vi "Search#OfTest.vi"(8 "TestStatusPath":path, 11 "MatchedSerialNumber":string) -> (3 "#OfTest":i32)   [LabVIEW 2011]
panel:
  out "#OfTest":string
  out "Status":string
  out "DateTime":string
  out "SerialNumber":string
  out "text":string
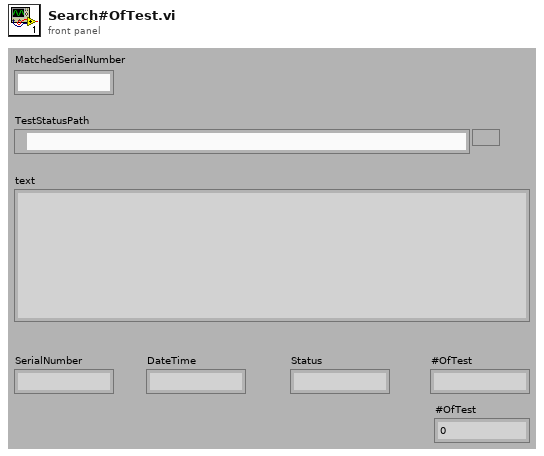
[diagram p1: front panel]
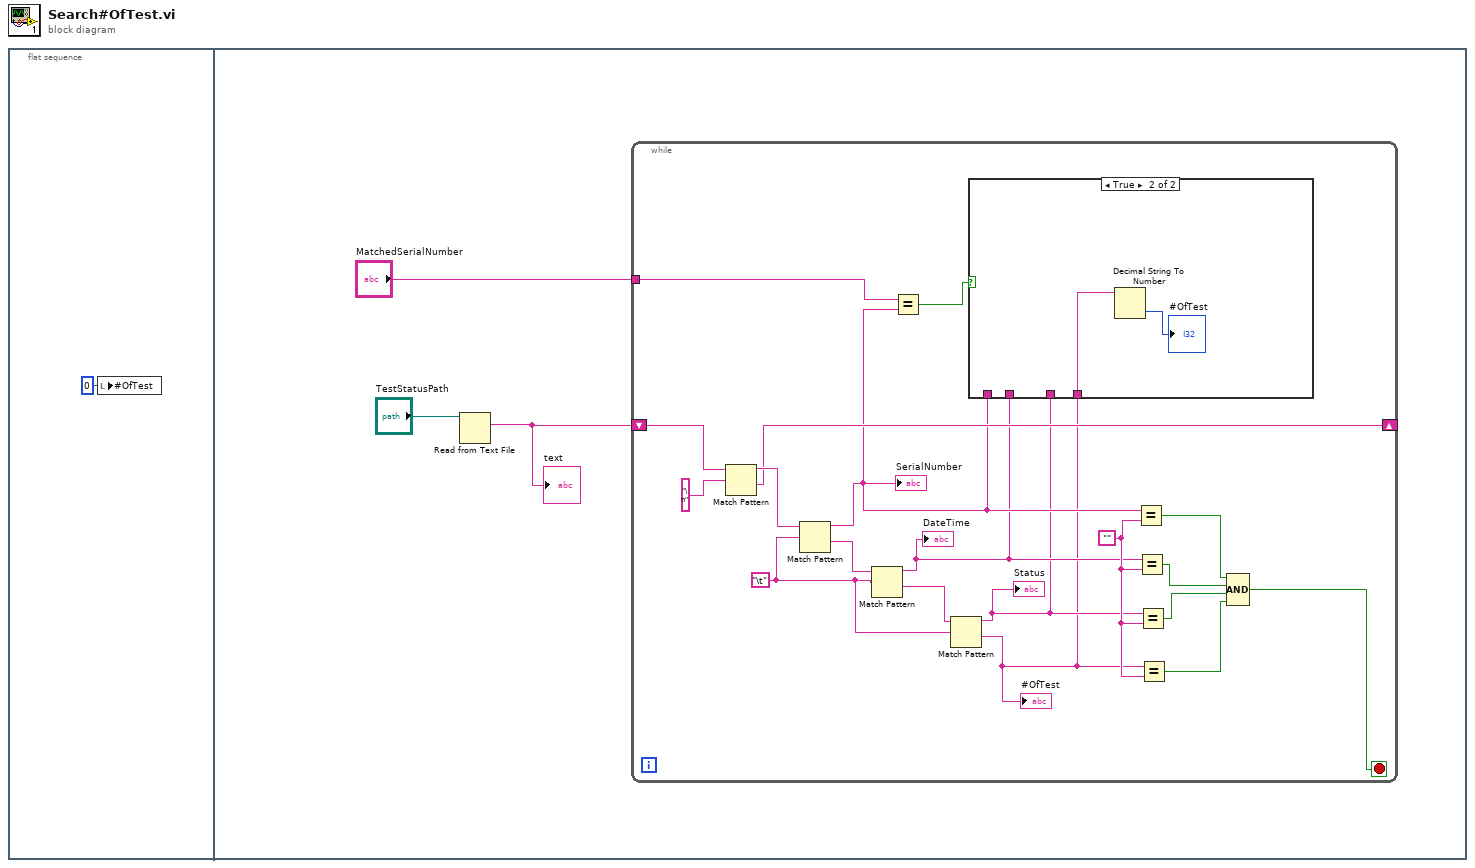
[diagram p0: block diagram]
diagram:
  n1 = flat-sequence {
    frame #0 {
      n2 = local write "#OfTest"(0 ("#OfTest")) -> ()
    }
    frame #1 {
      n3 = Read from Text File(file (use dialog)="TestStatusPath") -> (text=w4:string)  [unwired: 1 in, 5 out]
      "text" <- w4
      n4 = while {
        shift-right: [w11] -> _
        shift-left: w4 -> [w23]
        tunnel: "MatchedSerialNumber" -> [w10]
        stop <- w13 stop-if-true
        w18 = ""
        w19 = "\t"
        n5 = Match Pattern(string=w23, regular expression="\n") -> (before substring=w12:string, after substring=w11:string)  [unwired: 3 out]
        n6 = Match Pattern(string=w12, regular expression=w19) -> (before substring=w8:string, after substring=w21:string)  [unwired: 3 out]
        "SerialNumber" <- w8
        n7 = Match Pattern(string=w21, regular expression=w19) -> (before substring=w7:string, after substring=w20:string)  [unwired: 3 out]
        "DateTime" <- w7
        n8 = Equal?(x=w10, y=w8) -> (x = y?=w9:bool)
        n9 = Match Pattern(string=w20, regular expression=w19) -> (before substring=w6:string, after substring=w5:string)  [unwired: 3 out]
        "Status" <- w6
        "#OfTest" <- w5
        n10 = case shown="True" w9 {
          tunnel: w8 -> [_ _]
          tunnel: w7 -> [_ _]
          tunnel: w6 -> [_ _]
          tunnel: w5 -> [_ w24]
          frame False {
          }
          frame True {
            n11 = Decimal String To Number(string=w24) -> (number=→"#OfTest":i32)  [unwired: 3 out]
          }
        }
        n12 = Equal?(x=w8, y=w18) -> (x = y?=w17:bool)
        n13 = Equal?(x=w7, y=w18) -> (x = y?=w16:bool)
        n14 = Equal?(x=w6, y=w18) -> (x = y?=w15:bool)
        n15 = Equal?(x=w5, y=w18) -> (x = y?=w14:bool)
        n16 = Compound Arithmetic op=AND(w17, w16, w15, w14) -> (w13:bool)
      }
    }
  }
